vi "Write Command to Transfer Group.vi"(8 "error in (no error)":errorcluster, 9 "Command":T1=enum."Receive", 10 "Transfer Group":refnum<class "DSF.Engine.Transfer Group.lvclass">, 11 "Transceiver Interface in":refnum<class "Transceiver Interface.lvclass">) -> (0 "error out":errorcluster, 3 "Transceiver Interface out":refnum<class "Transceiver Interface.lvclass">)   [LabVIEW 2017, in "Data Sharing Framework Engine.lvlib" / "Transceiver Interface.lvclass"]
uses:
  Transceiver Interface.lvclass
  C:/github/data-sharing-framework/Source/Data Sharing Framework Core/Engine/Interfaces/Engine Interface/Engine Interface.lvclass
  old/dsf core/Source/Engine/Classes/Transfer/DSF.Engine.Transfer Group.lvclass
  Command.ctl
  old/dsf core/Source/Engine/Classes/Transfer/DSF.Engine.Transfer Group.lvclass/DSF.Engine.Transfer Group.ctl
  Timing/Engine Timing.lvclass/Engine Timing.ctl
  Command Data.ctl
  Command Parameters.ctl
  Engine Interface/Engine Interface.lvclass/Engine Interface.ctl
  Debug/Debug Flags FIFO/Debug Flags FIFO.lvclass/Debug Flags FIFO.ctl
  Write Transceiver Command.vi
  Write Command.vi
  Engine Interface/Get Command FIFO.vi
  Engine Interface/Write 16B RT FIFO.vi
  Engine Interface/Get Debug Flags.vi
  Debug/Debug Flags FIFO/Get Infinite Timeouts.vi
  Timing/Engine Timing.lvclass
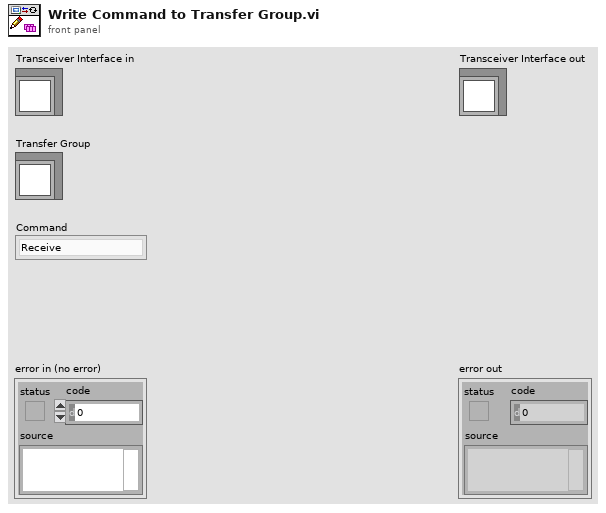
[diagram p1: front panel]
types:
  T1 = typedef "Data Sharing Framework Engine.lvlib/Transceiver Interface.lvclass/Command.ctl" = enum8{"Set Base Pointer", "Receive", "Transmit", "Shutdown"}
  T2 = cluster{"Transfer Group ID":i32, "unused":i32, "Transfer Group iteration":u64}
  T3 = typedef "Data Sharing Framework Engine.lvlib/Transceiver Interface.lvclass/Command Parameters.ctl" = cluster{"arg1":u64, "arg2":u64}
  T4 = typedef "Data Sharing Framework Engine.lvlib/Transceiver Interface.lvclass/Command Data.ctl" = cluster{"Command":T1, "Command Parameters":T3}
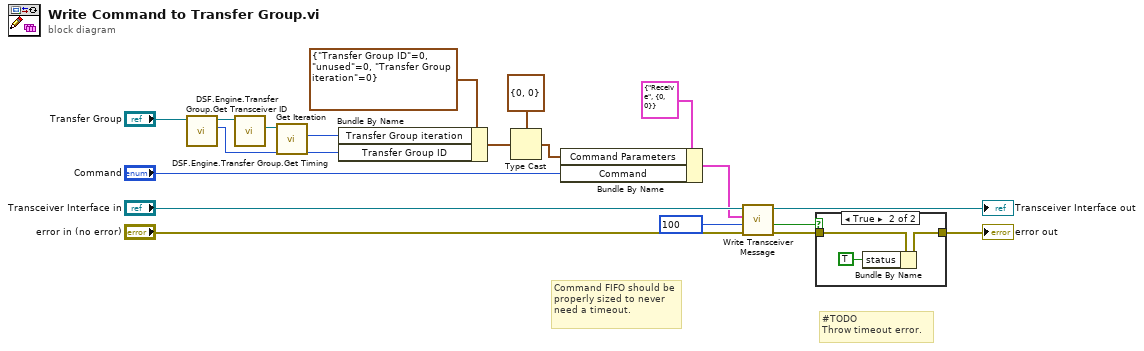
[diagram p0: block diagram]
diagram:
  # "Command FIFO should be properly sized to never need a timeout."
  # "#TODO\nThrow timeout error."
  n1 = call "DSF.Engine.Transfer Group.Get Transceiver ID.vi"("Transfer Group in"="Transfer Group") -> ("transceiver id"=w12:i32, "Transfer Group out"=w11:refnum<class "DSF.Engine.Transfer Group.lvclass">)  [unwired: 9 in]
  n2 = call "DSF.Engine.Transfer Group.Get Timing.vi"("Transfer Group in"=w11) -> ("Timing"=w10:refnum<class "Engine Timing.lvclass">)  [unwired: 9 in, 1 out]
  n3 = call "Get Iteration.vi"("Timing in"=w10) -> ("Iteration"=w9:u64)  [unwired: 9 in, 1 out]
  n4 = Bundle By Name(cluster=T2 {"Transfer Group ID"=0, "unused"=0, "Transfer Group iteration"=0}, "Transfer Group iteration"=w9, "Transfer Group ID"=w12) -> (w13:T2)
  n5 = Type Cast(type=T3 {"arg1"=0, "arg2"=0} ("Command Parameters"), x=w13) -> (*(type *) &x=w15:T3)
  n6 = Bundle By Name(cluster=T4 {"Command"=enum."Receive", "Command Parameters"={"arg1"=0, "arg2"=0}} ("command"), "Command Parameters"=w15, "Command"="Command") -> (w1:T4)
  n7 = call-poly "Write Transceiver Message.vi"("error in (no error)"="error in (no error)", "timeout in ms (0)"=100, "command"=w1, "Transceiver Interface in"="Transceiver Interface in") -> ("error out"=w7:errorcluster, "timed out?"=w8:bool, "Transceiver Interface out"=→"Transceiver Interface out":refnum<class "Transceiver Interface.lvclass">)  [unwired: 5 in]
  n8 = case shown="True" w8 {
    tunnel: w7 -> [w20 w23]
    tunnel: [w20 w22] -> w6
    frame False {
    }
    frame True {
      n9 = Bundle By Name(cluster=w23, "status"=TRUE) -> (w22:errorcluster)
    }
  }
  "error out" <- w6
